vi "Experiment_Resonator_open.vi"() -> ()   [LabVIEW 2009]
uses:
  <vilib>/imath/engines/lvmath2/RunTimeEngine/ErrorHandling/NIMS_Finalize Error.vi
  <vilib>/imath/engines/lvmath2/RunTimeEngine/Parser/MC_Version.vi
  <vilib>/imath/engines/lvmath2/RunTimeEngine/Managers/WorkSpace/UID Generator.vi
  <vilib>/imath/engines/lvmath2/RunTimeEngine/NodeEndStatement/NIMS_NodeEndStatement_Output.vi
  <instcachedir>/0/NIMS_NodeEndStatement_Output_B70DDD75627E4997AAE11E9955EDAA25.lvgen/NIMS_NodeEndStatement_Output_B70DDD75627E4997AAE11E9955EDAA25_001.vi
  <instcachedir>/0/NIMS_NodeEndStatement_Output_B70DDD75627E4997AAE11E9955EDAA25.lvgen/NIMS_NodeEndStatement_Output_B70DDD75627E4997AAE11E9955EDAA25_000.vi
  <vilib>/imath/engines/lvmath2/RunTimeEngine/Managers/SymbolTable/Clear UID.vi
  <vilib>/imath/engines/lvmath/Functions/Error Handling/MergeErrorsWrapper.vi
  <vilib>/imath/engines/lvmath2/RunTimeEngine/LocalVariableDefStatement/MC_LocalVariableDefStatement_Display.vi
  <vilib>/imath/engines/lvmath2/RunTimeEngine/RunTimeType/NIMS_RunTimeType_From StrictType (excl LVString).vi
  <vilib>/imath/engines/lvmath2/RunTimeEngine/RangeToken/NIMS_Range.vi
  <instcachedir>/0/NIMS_Range_6D647EC16A744C98B5DE1D649A2D648D.lvgen/NIMS_Range_6D647EC16A744C98B5DE1D649A2D648D_001.vi
  <vilib>/imath/engines/lvmath2/RunTimeEngine/VariableToken/NIMS_VariableToken_CondDefined.vi
  <instcachedir>/0/NIMS_VariableToken_CondDefined_5641E79000FB4D628475532441475385.lvgen/NIMS_VariableToken_CondDefined_5641E79000FB4D628475532441475385_001.vi
  <vilib>/imath/engines/lvmath/Functions/Error Handling/error.ctl
  <vilib>/imath/engines/lvmath/Functions/Error Handling/MC_Mask_Errors.vi
  <vilib>/imathl/engines/lvmath/Functions/Error Handling/Create Error.vi
  <vilib>/imath/engines/lvmath2/RunTimeEngine/ReplaceToken/NIMS_Replace - V(S)=S.vi
  <instcachedir>/0/NIMS_Replace - V(S)=S_670A9E0533664C1D848C8E58B3321B6A.lvgen/NIMS_Replace - V(S)=S_670A9E0533664C1D848C8E58B3321B6A_000.vi
  <vilib>/imath/engines/lvmath2/RunTimeEngine/ReplaceToken/NIMS_Replace - Size Check _(_)=S.vi
  <instcachedir>/0/NIMS_Replace - Size Check _(_)=S_8596181D73404097BAB9CBB006194BB0.lvgen/NIMS_Replace - Size Check _(_)=S_8596181D73404097BAB9CBB006194BB0_001.vi
  <vilib>/imath/engines/lvmath2/RunTimeEngine/ReplaceToken/NIMS_Replace - Check Linear.vi
  <instcachedir>/0/NIMS_Replace - Check Linear_9243CBB174894FF6977027453DA6955E.lvgen/NIMS_Replace - Check Linear_9243CBB174894FF6977027453DA6955E_001.vi
  <vilib>/imath/engines/lvmath2/RunTimeEngine/VariableToken/NIMS_VariableToken_CondDefinedDefinedByReplace.vi
  <instcachedir>/0/NIMS_VariableToken_CondDefinedDefinedByReplace_D162CFFC24174562A9FEA619A91E1A56.lvgen/NIMS_VariableToken_CondDefinedDefinedByReplace_D162CFFC24174562A9FEA619A91E1A56_001.vi
  <vilib>/imath/engines/lvmath2/RunTimeEngine/CommandStatement/MC_CommandStatement_break.vi
  <vilib>/imath/engines/lvmath2/RunTimeEngine/Managers/SymbolTable/NIMS_WorkSpace.lvlib
panel:
  out "error out":errorcluster
  out "error out":errorcluster
  in  "?":enum32{"TRANSMISSION LINE DEMONSTRATION"}(tab)
  out "?":cluster{dbl[]}[](graph)
  in  "Delay Time (s)":dbl min=0.0 max=10.0 step=0.005
  out "?":errorcluster
  in  "HELP FOR TLD":bool
  in  "?":enum32{"SOURCE"}(tab)
  out "?":errorcluster
  in  "Frequency of carrier wave(Hz)":i8(slide) scale=1.0..4.0
  out "?":dbl[](graph)
  in  "Voltage":dbl(knob) scale=0.0..10.0 scale format="%#_10g"
  in  "HELP FOR SOURCE":bool
  # "Transmisson line demonstrator"
  # "Function generator"
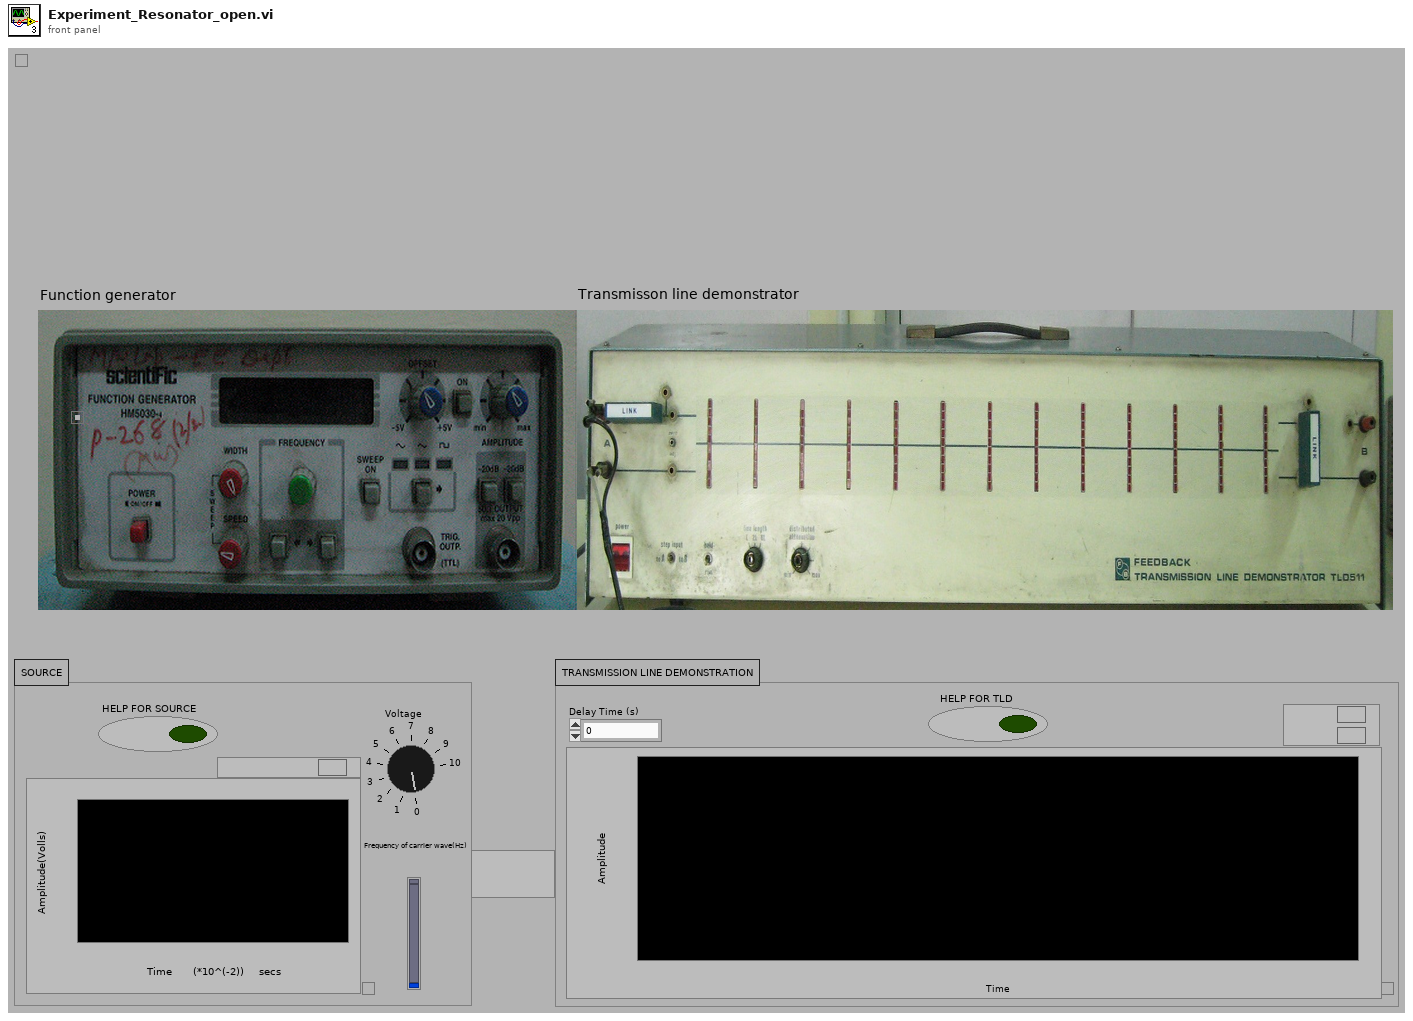
[diagram p1: front panel]
types:
  T1 = typedef "error.ctl" = enum16{"No Error", "Problem", "Unused002", "Incorrect number of parameters", "Function not defined for non-numeric types", "Unused005", "Function only defined for character arrays", "Function not defined for boolean, character, or single precision", "Function not defined for complex types", "Not a valid operation", "Inputs must be scalar", "Input matrices are not the same size", "Unused012", "Input matrices must be nonnegative integers of the same type", "Arguments must be non-negative integers less than bitmax", "Number to complement must be less than 2^N", "Bit to get is outside range", "Bit to set is outside range", "Input must be real type ", "At least one parameter must be scalar", "Unused020", "Function not defined for\nhigher dimensional matrices.", "Invalid attributes", "Wrong Type of Input Arguments", "Wrong Argument Option", "Unused025", "Indices must be real positive integers", "Unused027", "Number of elements must be the same for indices and values", "Unused029", "Cannot resize a 2D matrix with a linear index", "Unknown variable or symbol", "Indices out of range", "Empty matrix deletion can not be used with two indices", "Number of rows and columns must be the same for indices and values.", "Complex cannot be converted to Boolean", "Char cannot be converted to Boolean", "int64 cannot be converted to Boolean", "uint64 cannot be converted to Boolean", "Unused039", "Unused040", "All rows must have the same number of columns", "Incompatible types", "Invalid matrix dimensions", "Dimension must be 1 or 2", "Base must be an integer between 2 and 36", "Invalid input", "Square matrix required", "Function 'timerstart' must be called before 'timerstop'", "Arguments must be positive real", "Step must not be zero", "Wrong number of input arguments", "Wrong number of output arguments", "Unused053", "Input scalar must be >= 0", "Input scalar must be positive", "Input scalar must not be 0", "Input scalar must be in range [0,1]", "Unused058", "Input must be a vector", "Unused060", "Empty vector error", "All elements must be in domain [-1,1]", "All real elements of input vector must be >= 0", "All elements of input vector must be positive", "Values of input vectors are not compatible", "Unused066", "Input vector must be an increasing vector", "Unused068", "Unused069", "Lenths of two input vectors are not compatible", "Unused071", "Empty matrix error", "Unused073", "Unused074", "Unused075", "Unused076", "Unused077", "Size of input matrix is incompatible with input size", "Invalid format specifier", "Unused080", "Unused081", "Unused082", "Unused083", "Unused084", "Unused085", "RunTime: MathScript could not be compiled", "Unknown function", "Only scalars and strings supported", "Unused089", "Unused090", "Range is too large", "End used without variable", "Function not available (RTE)", "Custom user error", "Arguments must be integers less than bitmax", "Shared library not found", "Header file not found", "Shared library already loaded", "Shared library not loaded", "Shared library function not found", "Shared library string return problem", "Problem calling shared library function", "Problem loading shared library from OS", "Problem parsing shared library header file", "Shared library incompatible types", "Shared library unsupported return type", "Shared library function not exported", "Shared library unsupported input type", "Problem unloading shared library from OS", "Function only available from UI", "Invalid function specified in argument", "An internal error has occurred", "Invalid object", "Invalid property", "Read-only property", "A break command has occurred", "A continue command has occurred", "A return command has occurred", "ode: times parameter invalid", "Unused120", "Function not found in file", "Reserved keyword cannot be defined as variable", "Reserved keyword cannot be defined as a function or script", "Arguments must be string literals", "Function not supported on this platform", "All columns must have the same number of rows", "Function ignored in RTE warning", "Cannot use : as a parameter that is not a variable", "Output can't be coerced to requested type", "Function not supported on current target", "Variable dependent on an unwired function input", "Unused132", "Unused133", "Unused134", "Unused135", "Unused136", "Unused137", "Unused138", "Unused139", "Unused140", "Unused141", "Unused142", "Unused143", "Unused144", "Unused145", "Unused146", "MathScript parser DLL missing", "MathScript requires LabVIEW Full", "MathScript license is invalid or missing"}
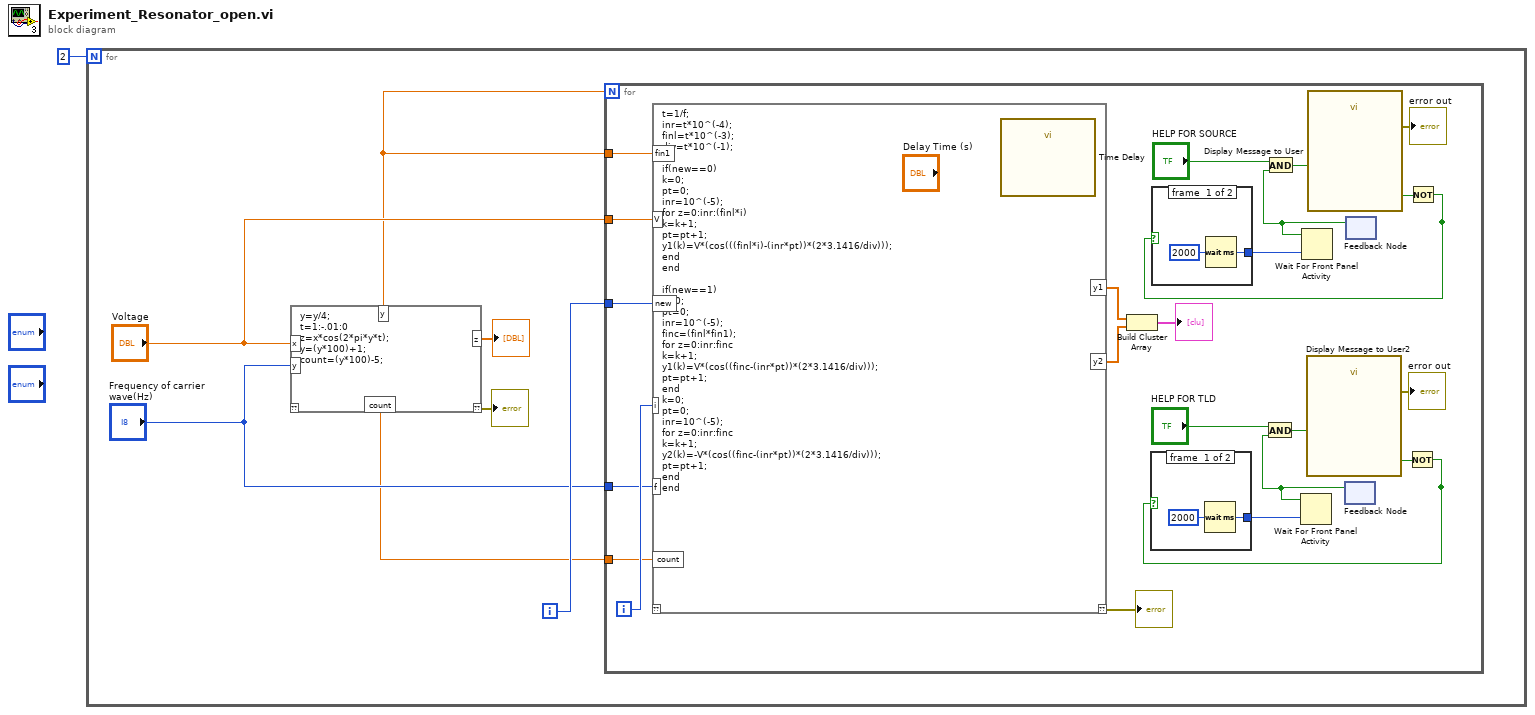
[diagram p0: block diagram]
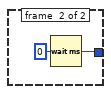
[diagram p2: hidden frame]
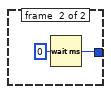
[diagram p3: hidden frame]
diagram:
  n1 = for {
    N: 2 -> [_]
    i -> [w8]
    n2 = mathscript code="y=y/4;\nt=1:-.01:0\nz=x*cos(2*pi*y*t);\ny=(y*100)+1;\ncount=(y*100)-5;"("x"="Voltage", "y"="Frequency of carrier wave(Hz)") -> ("??"=→"?":errorcluster, "z"=→"?":dbl[], "y"=w2:dbl, "count"=w3:dbl)  [unwired: 1 in]
    n3 = for {
      N: w2 -> [_]
      tunnel: w8 -> [w118]
      tunnel: "Voltage" -> [w117]
      tunnel: "Frequency of carrier wave(Hz)" -> [w116]
      tunnel: w3 -> [w115]
      tunnel: w2 -> [w110]
      i -> [w119]
      n4 = mathscript code="t=1/f;\ninr=t*10^(-4);\nfinl=t*10^(-3);\ndiv=t*10^(-1);\n\nif(new==0)\nk=0;\npt=0;\ninr=10^(-5);\nfor z=0:inr:(finl*i)\nk=k+1;\npt=pt+1;\ny1(k)=V*(cos(((finl*i)-(inr*pt))*(2*3.1416/div)));\nend\nend\n\nif(new==1)\nk=0;\npt=0;\ninr=10^(-5);\nfinc=(finl*fin1);\nfor z=0:inr:finc\nk=k+1;\ny1(k)=V*(cos((finc-(inr*pt))*(2*3.1416/div)));\npt=pt+1;\nend\nk=0;\npt=0;\ninr=10^(-5);\nfor z=0:inr:finc\nk=k+1;\ny2(k)=-V*(cos((finc-(inr*pt))*(2*3.1416/div)));\npt=pt+1;\nend\nend"("i"=w119, "new"=w118, "V"=w117, "f"=w116, "count"=w115, "fin1"=w110) -> ("??"=→"?":errorcluster, "y1"=w113:dbl[], "y2"=w112:dbl[])  [unwired: 1 out]
      n5 = call "Time Delay"("Delay Time (s)"="Delay Time (s)") -> ()  [unwired: 1 in, 10 out]
      n6 = Build Cluster Array(w113, w112) -> (→"?":cluster{dbl[]}[])
      n7 = feedback #1() -> (w99:bool)  [unwired: 1 in]
      n8 = And(x="HELP FOR TLD", y=w99) -> (x .and. y?=w100:bool)
      n9 = call "Display Message to User2"("Enable"=w100) -> ("error out"=→"error out":errorcluster, "CLOSE"=w98:bool)  [unwired: 2 in, 7 out]
      n10 = feedback #2() -> (w106:bool)  [unwired: 1 in]
      n11 = And(x="HELP FOR SOURCE", y=w106) -> (x .and. y?=w107:bool)
      n12 = call "Display Message to User"("Enable"=w107) -> ("error out"=→"error out":errorcluster, "CLOSE"=w105:bool)  [unwired: 2 in, 7 out]
      n13 = Not(x=w98) -> (.not. x?=w96:bool)
      n14 = case shown="False" w96 {
        tunnel: [w120 w122] -> w95
        frame #0 {
          n15 = Wait (ms)(milliseconds to wait=u32 2000) -> (millisecond timer value=w120:u32)
        }
        frame #1 {
          n16 = Wait (ms)(milliseconds to wait=u32 0) -> (millisecond timer value=w122:u32)
        }
      }
      n17 = Wait For Front Panel Activity(1:w95, 3:w99) -> ()  [unwired: 1 in, 1 out]
      n18 = Not(x=w105) -> (.not. x?=w103:bool)
      n19 = case shown="False" w103 {
        tunnel: [w124 w126] -> w102
        frame #0 {
          n20 = Wait (ms)(milliseconds to wait=u32 2000) -> (millisecond timer value=w124:u32)
        }
        frame #1 {
          n21 = Wait (ms)(milliseconds to wait=u32 0) -> (millisecond timer value=w126:u32)
        }
      }
      n22 = Wait For Front Panel Activity(1:w102, 3:w106) -> ()  [unwired: 1 in, 1 out]
    }
  }
